vi "氨氮电源命令.vi"(10 "通电/断电":bool, 11 "队列":refnum<queue>) -> (3 "队列输出":refnum<queue>)   [LabVIEW 2016, in "环境动力监测库.lvlib" / "V电源管理库.lvlib"]
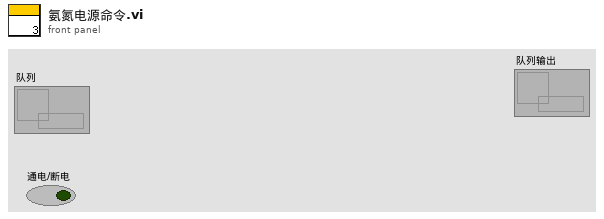
[diagram p1: front panel]
types:
  T1 = cluster{"状态":cluster{"R0":i16, "R1":i16, "R2":i16, "R3":i16, "R4":i16, "R5":i16, "R6":i16, "R7":i16, "R8":i16, "R9":i16, "R10":i16, "R11":i16, "R12":i16, "R13":i16, "R14":i16, "R15":i16, "R16":i16, "R17":i16, "R18":i16, "R19":i16, "R20":i16, "R21":i16, "R22":i16, "R23":i16, "R24":i16, "R25":i16, "R26":i16, "R27":i16, "R28":i16, "R29":i16, "R30":i16, "R31":i16, "R32":i16, "R33":i16, "R34":i16, "R35":i16, "R36":i16, "R37":i16, "R38":i16, "R39":i16, "R40":i16, "R41":i16, "R42":i16, "R43":i16, "R44":i16, "R45":i16, "R46":i16, "R47":i16, "R48":i16, "R49":i16, "R50":i16, "R51":i16, "R52":i16, "R53":i16, "R54":i16, "R55":i16, "R56":i16, "R57":i16, "R58":i16, "R59":i16, "R60":i16, "R61":i16, "R62":i16, "R63":i16, "R64":i16, "R65":i16, "R66":i16, "R67":i16, "R68":i16, "R69":i16}, "输入状态":bool[], "输出状态":bool[], "报警簇":bool[], "参数设置":cluster{"R100":i16, "R101":i16, "R102":i16, "R103":i16, "R104":i16, "R105":i16, "R106":i16, "R107":i16, "R108":i16, "R109":i16, "R110":i16, "R111":i16, "R112":i16, "R113":i16, "R114":i16, "R115":i16, "R116":i16, "R117":i16, "R118":i16, "R119":i16, "R120":i16, "R121":i16, "R122":i16, "R123":i16, "R124":i16}, "转换值":cluster{"AD0":sgl, "AD1":sgl, "AD2":sgl, "AD3":sgl, "AD4":sgl, "AD5":sgl}, "看门狗启用":bool, "氨氮模块名称":string, "总磷模块名称":string, "采配水模块类型":enum16{"V1", "V2", "V3", "V4", "室内V1", "室内V2"}}
  T2 = cluster{"命令":string, "data":cluster{"starting address":u16, "coil values":bool[]}}
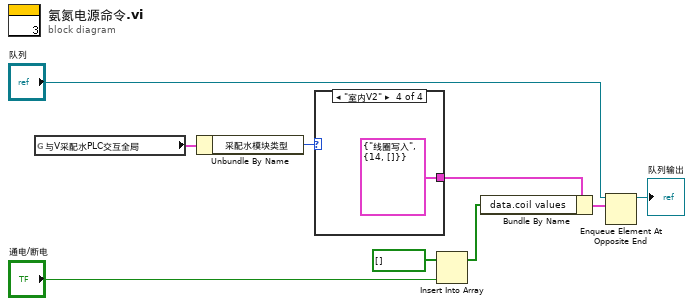
[diagram p0: block diagram]
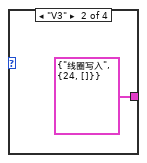
[diagram p3: hidden frame]
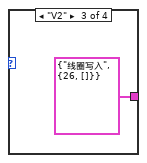
[diagram p4: hidden frame]
diagram:
  n1 = global read "外部交互全局变量.vi" "与V采配水PLC交互全局"() -> (w3:T1)
  n2 = Unbundle By Name(w3) -> ("采配水模块类型"=w2:enum16{"V1", "V2", "V3", "V4", "室内V1", "室内V2"})
  n3 = case shown="\"室内V2\"" w2 {
    tunnel: [_ T2 {"命令"="线圈写入", "data"={"starting address"=24, "coil values"=[]}} ("元素") T2 {"命令"="线圈写入", "data"={"starting address"=26, "coil values"=[]}} ("元素") T2 {"命令"="线圈写入", "data"={"starting address"=14, "coil values"=[]}} ("元素")] -> w1
    frame "V1", Default {
    }
    frame "V3" {
    }
    frame "V2" {
    }
    frame "室内V2" {
    }
  }
  n4 = Insert Into Array(array=bool[] [] ("data.coil values"), new element="通电/断电") -> (w5:bool[])  [unwired: 1 in]
  n5 = Bundle By Name(cluster=w1, "data.coil values"=w5) -> (w9:T2)
  n6 = Enqueue Element At Opposite End(queue="队列", element=w9) -> (queue out=→"队列输出":refnum<queue>)  [unwired: 2 in, 2 out]
